vi "SignalIntegrator.vi"(4 "Ts":dbl, 8 "Reset":bool, 11 "x":dbl) -> (3 "y":dbl)   [LabVIEW 2019]
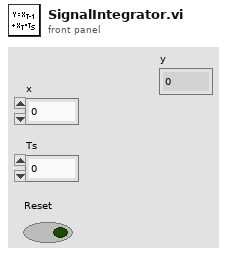
[diagram p1: front panel]
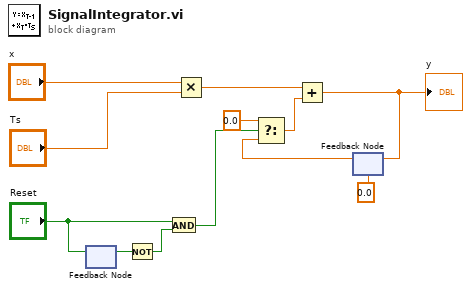
[diagram p0: block diagram]
diagram:
  n1 = feedback #1() -> (w7:bool)  [unwired: 1 in]
  n2 = feedback-in #1 ("2")("Reset") -> ()
  n3 = Not(x=w7) -> (.not. x?=w5:bool)
  n4 = And(x="Reset", y=w5) -> (x .and. y?=w2:bool)
  n5 = Multiply(x="x", y="Ts") -> (x*y=w11:dbl)
  n6 = feedback #2(0.0 ("Constant")) -> (w3:dbl)
  n7 = Select(t=0.0, s=w2, f=w3) -> (s? t:f=w4:dbl)
  n8 = Add(x=w11, y=w4) -> (x+y=w12:dbl)
  "y" <- w12
  n9 = feedback-in #2 ("2")(w12) -> ()
